vi "Dump Holt Memory.vi"(8 "error IO":errorcluster, 11 "FPGA Interface":refnum<class "FPGA Interface.lvclass">) -> (0 "error out":errorcluster, 3 "appended array":string[][](array[string]))   [LabVIEW 2016]
uses:
  Utilities/FPGA Interface/FPGA Interface.lvclass
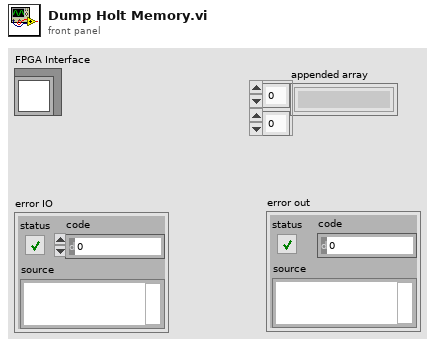
[diagram p1: front panel]
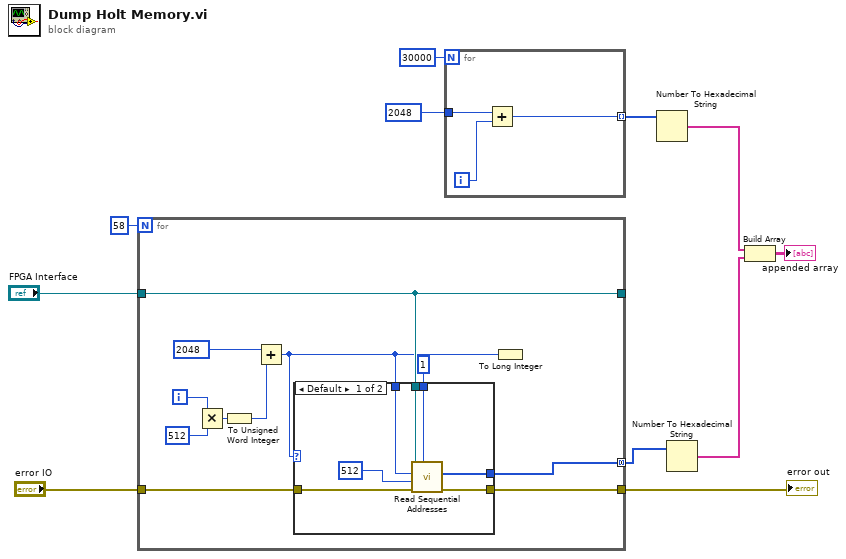
[diagram p0: block diagram]
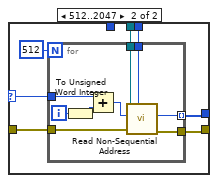
[diagram p2: hidden frame]
diagram:
  n1 = for {
    N: 58 -> [_]
    tunnel: "error IO" -> [w22]
    tunnel: [w13] -> w8
    tunnel: "FPGA Interface" -> [w16]
    tunnel: [w16] -> _
    tunnel: [w14] -> w7 mode=concatenating
    i -> [w21]
    n2 = Multiply(x=w21, y=512) -> (x*y=w20:i32)
    n3 = To Unsigned Word Integer(number=w20) -> (unsigned 16bit integer=w19:u16)
    n4 = Add(x=u16 2048 ("Address"), y=w19) -> (x+y=w15:u16)
    n5 = case shown="Default" w15 {
      selector: w15 -> [_ w30]
      tunnel: w22 -> [w29 w36]
      tunnel: w15 -> [w28 _]
      tunnel: [w27 w35] -> w13
      tunnel: u8 1 ("Component ID") -> [w26 w33]
      tunnel: w16 -> [w25 w32]
      tunnel: [w24 w34] -> w14
      frame Default {
        n6 = call-dynamic "Read Sequential Addresses.vi"("Target IC (1-8)"=w26, "error in (no error)"=w29, "Addresses to Read"=u16 512 ("y"), "Starting Address"=w28, "FPGA Interface in"=w25) -> ("error out"=w27:errorcluster, "Data"=w24:u16[])  [unwired: 5 in]
      }
      frame 512..2047 {
        n7 = for {
          N: 512 -> [_]
          tunnel: w36 -> [w45]
          tunnel: [w44] -> w35
          tunnel: [w43] -> w34 mode=indexing
          tunnel: w33 -> [w42]
          tunnel: w32 -> [w41]
          tunnel: w30 -> [w40]
          i -> [w39]
          n8 = To Unsigned Word Integer(number=w39) -> (unsigned 16bit integer=w37:u16)
          n9 = Add(x=w40, y=w37) -> (x+y=w38:u16)
          n10 = call-dynamic "Read Non-Sequential Address.vi"("Target IC (1-8)"=w42, "error in (no error)"=w45, "Address"=w38, "FPGA Interface in"=w41) -> ("error out"=w44:errorcluster, "Data"=w43:u16)  [unwired: 6 in]
        }
      }
    }
    n11 = To Long Integer(number=w15) -> ()  [unwired: 1 out]
  }
  "error out" <- w8
  n12 = for {
    N: 30000 -> [_]
    tunnel: u16 2048 ("Address") -> [w48]
    tunnel: [w46] -> w5 mode=indexing
    i -> [w47]
    n13 = Add(x=w48, y=w47) -> (x+y=w46:i32)
  }
  n14 = Number To Hexadecimal String(2:w5) -> (0:w4:string[])  [unwired: 1 in]
  n15 = Number To Hexadecimal String(2:w7) -> (0:w3:string[])  [unwired: 1 in]
  n16 = Build Array(w4, w3) -> (→"appended array":string[][])
